vi "Init.vi"(8 "error in (no error)":errorcluster, 10 "Price":dbl, 11 "Shower in":refnum<class "Shower.lvclass">) -> (0 "error out":errorcluster, 3 "Shower out":refnum<class "Shower.lvclass">)   [LabVIEW 2019, in "Shower.lvclass"]
uses:
  Shower.lvclass
  Furniture.lvclass
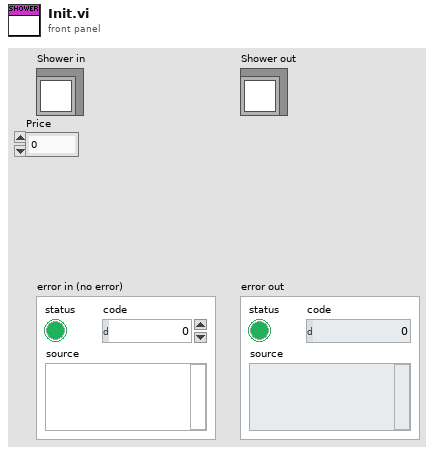
[diagram p1: front panel]
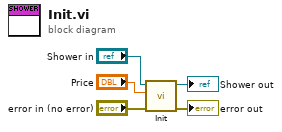
[diagram p0: block diagram]
diagram:
  n1 = call-parent "Init.vi"("error in (no error)"="error in (no error)", "Price"="Price", "Furniture in"="Shower in") -> ("error out"=→"error out":errorcluster, "Furniture out"=→"Shower out":refnum<class "Shower.lvclass">)  [unwired: 7 in]
